vi "FindPeaks_old.vi"(11 "subarray":cdb[](array[numeric])) -> (1 "indicies":i32[](array[numeric]), 3 "Array in":dbl[](graph))   [LabVIEW 2024]
panel:
  out "Array in 2":dbl[](graph)
  out "XY Graph":cluster{i32[], "Array in":dbl[]}[](graph)
  out "amplitude":dbl
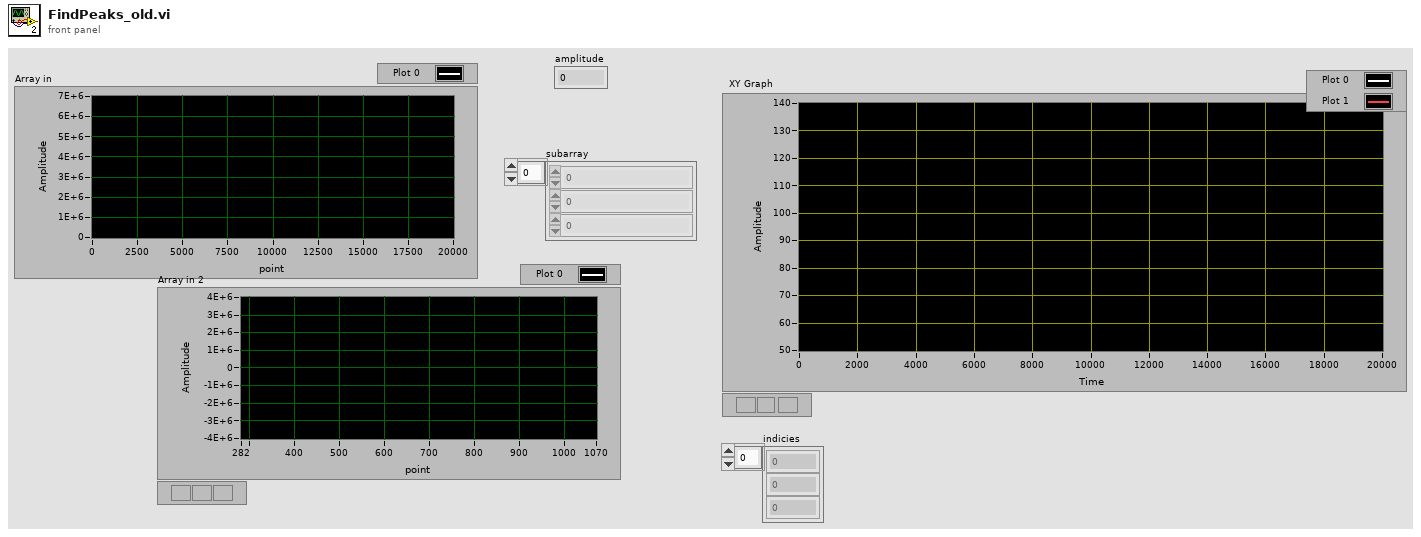
[diagram p1: front panel]
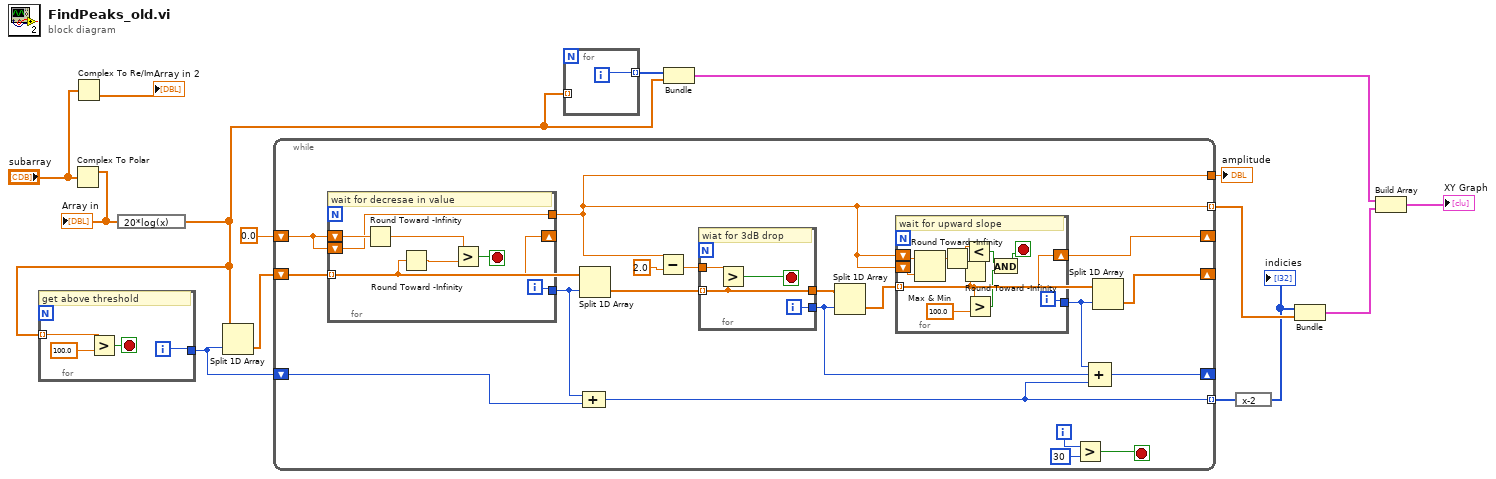
[diagram p0: block diagram]
diagram:
  n1 = Complex To Polar(r * e^(i*theta)="subarray") -> (r=w8:dbl[])  [unwired: 1 out]
  "Array in" <- w8
  n2 = Complex To Re/Im(x + iy="subarray") -> (y=→"Array in 2":dbl[])  [unwired: 1 out]
  n3 = expression code="20*log(x)"(w8) -> (w5:dbl[])
  n4 = for {
    tunnel: w5 -> [w18] mode=indexing
    tunnel: [w19] -> w4
    i -> [w19]
    stop <- w16 stop-if-true
    # "get above threshold"
    n5 = Greater?(x=w18, y=100.0) -> (0:w16:bool)
  }
  n6 = Split 1D Array(array=w5, index=w4) -> (second subarray=w6:dbl[])  [unwired: 1 out]
  n7 = while {
    tunnel: [w21] -> w15
    shift-right: [w29] -> _
    shift-left: w6 -> [w37]
    shift-right: [w32] -> _
    shift-left: 0.0 -> [w20]
    shift-right: [w28] -> _
    shift-left: w4 -> [w23]
    tunnel: [w22] -> w3 mode=indexing
    tunnel: [w21] -> w11 mode=indexing
    i -> [w27]
    stop <- w25 stop-if-true
    n8 = for {
      tunnel: w37 -> [w55] mode=indexing
      shift-right: [w55] -> _
      shift-left: w20 -> [w56]
      tunnel: [w58] -> w24
      tunnel: [w53] -> w21
      shift-left: w20 -> [w53]
      i -> [w58]
      stop <- w59 stop-if-true
      # "wait for decresae in value"
      n9 = Round Toward -Infinity(1:w56) -> (0:w57:dbl)
      n10 = Round Toward -Infinity(1:w55) -> (0:w54:dbl)
      n11 = Greater?(x=w57, y=w54) -> (0:w59:bool)
    }
    n12 = Split 1D Array(array=w37, index=w24) -> (second subarray=w34:dbl[])  [unwired: 1 out]
    n13 = Compound Arithmetic op=ADD(w24, w23) -> (w22:i32)
    n14 = Subtract(x=w21, y=2.0) -> (x-y=w35:dbl)
    n15 = for {
      tunnel: w34 -> [w50] mode=indexing
      tunnel: w35 -> [w52]
      tunnel: [w50] -> _
      tunnel: [w51] -> w31
      i -> [w51]
      stop <- w49 stop-if-true
      # "wiat for 3dB drop"
      n16 = Greater?(x=w52, y=w50) -> (0:w49:bool)
    }
    n17 = Split 1D Array(array=w34, index=w31) -> (second subarray=w33:dbl[])  [unwired: 1 out]
    n18 = for {
      tunnel: w33 -> [w47] mode=indexing
      shift-right: [w47] -> w32
      shift-left: w21 -> [w41]
      tunnel: [w48] -> w30
      shift-left: w21 -> [w40]
      i -> [w48]
      stop <- w43 stop-if-true
      # "wait for upward slope"
      n19 = Max & Min(x=w41, y=w40) -> (max(x,y)=w42:dbl)  [unwired: 1 out]
      n20 = Round Toward -Infinity(1:w42) -> (0:w39:dbl)
      n21 = Round Toward -Infinity(1:w47) -> (0:w38:dbl)
      n22 = Less?(x=w39, y=w38) -> (x < y?=w45:bool)
      n23 = Greater?(x=w47, y=100.0) -> (0:w44:bool)
      n24 = And(x=w45, y=w44) -> (x .and. y?=w43:bool)
    }
    n25 = Greater?(x=w27, y=30) -> (0:w25:bool)
    n26 = Compound Arithmetic op=ADD(w30, w31, w22) -> (w28:i32)
    n27 = Split 1D Array(array=w33, index=w30) -> (second subarray=w29:dbl[])  [unwired: 1 out]
  }
  "amplitude" <- w15
  n28 = for {
    tunnel: [w60] -> w13 mode=indexing
    tunnel: w5 -> [_] mode=indexing
    i -> [w60]
  }
  n29 = Bundle(w13, w5) -> (w12:cluster{i32[], dbl[]})  [unwired: 1 in]
  n30 = expression code="x-2"(w3) -> (w2:i32[])
  "indicies" <- w2
  n31 = Bundle(w2, w11) -> (w10:cluster{i32[], dbl[]})  [unwired: 1 in]
  n32 = Build Array(w12, w10) -> (→"XY Graph":cluster{i32[], dbl[]}[])
